vi "Init VAR.vi"(10 "Simple VAR type args":T4={"ParameterName"="", "Index"=0, "DataType"=0, "DefaultValue"="", "AccessType"=enum."UNKNOWN", "PDOMappingType"=enum."NO"} {"DataType" items=["UNKNOWN", "BOOLEAN", "INTEGER8", "INTEGER16", "INTEGER32", "UNSIGNED8", "UNSIGNED16", "UNSIGNED32", "REAL32", "VISIBLE_STRING", "OCTET_STRING", "UNICODE_STRING", "TIME_OF_DAY", "TIME_DIFFERENCE", "DOMAIN", "INTEGER24", "REAL64", "INTEGER40", "INTEGER48", "INTEGER56", "INTEGER64", "UNSIGNED24", "UNSIGNED40", "UNSIGNED48", "UNSIGNED56", "UNSIGNED64", "PDO_COMMUNICATION_PARAMETER", "PDO_MAPPING", "SDO_PARAMETER", "IDENTITY"]}, 11 "OD Entry in":refnum<class "OD Entry.lvclass">) -> (3 "OD Entry out":refnum<class "OD Entry.lvclass">)   [LabVIEW 2024, in "EDS.lvlib" / "OD Entry.lvclass"]
doc: "Simple VAR type arguments"
uses:
  OD Entry.lvclass
  Data Type.ctl
  Access Type.ctl
  PDO Mapping Type.ctl
  OD Entry.lvclass/OD Entry.ctl
  EDS.lvlib
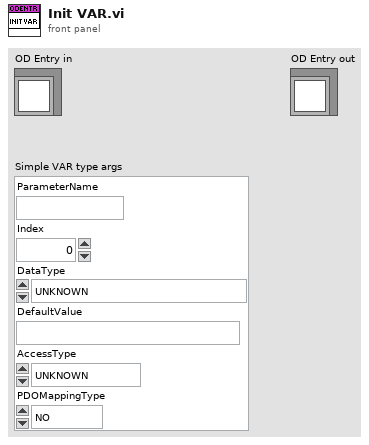
[diagram p1: front panel]
types:
  T1 = typedef "EDS.lvlib/Data Type.ctl" = u16
  T2 = typedef "EDS.lvlib/Access Type.ctl" = enum16{"rw", "ro", "wo", "rwr", "rww", "@const", "UNKNOWN"}
  T3 = typedef "EDS.lvlib/PDO Mapping Type.ctl" = enum16{"NO", "OPTIONAL", "RPDO", "TPDO", "@DEFAULT"}
  T4 = cluster{"ParameterName":string, "Index":u16, "DataType":T1, "DefaultValue":string, "AccessType":T2, "PDOMappingType":T3}
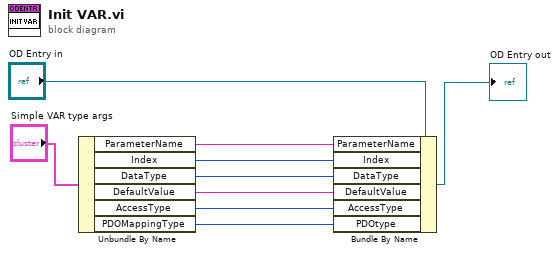
[diagram p0: block diagram]
diagram:
  n1 = Unbundle By Name("Simple VAR type args") -> ("ParameterName"=w6:string, "Index"=w5:u16, "DataType"=w4:T1, "DefaultValue"=w3:string, "AccessType"=w2:T2, "PDOMappingType"=w1:T3)
  n2 = Bundle By Name(cluster="OD Entry in", "ParameterName"=w6, "Index"=w5, "DataType"=w4, "DefaultValue"=w3, "AccessType"=w2, "PDOtype"=w1) -> (→"OD Entry out":refnum<class "OD Entry.lvclass">)
